vi "KeyDown.vi"(9 "Virtual Key":u8(ring)=65) -> ()   [LabVIEW 2020]
doc: "call keybd_event drom user32.dll library to generate the key down event on desired key"
uses:
  user32.dll
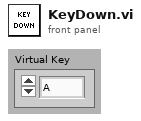
[diagram p1: front panel]
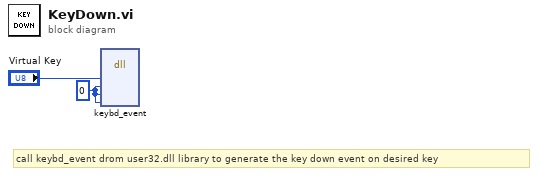
[diagram p0: block diagram]
diagram:
  w2 = u8 0 ("bScan")
  # "call keybd_event drom user32.dll library to generate the key down event on desired key"
  n1 = dll-call lib="user32.dll" fn="keybd_event"("bVk"="Virtual Key", "bScan"=w2, "dwFlags"=w2, "dwExtraInfo"=w2) -> ()  [unwired: 8 in, 2 out]
